vi "element_editor_methane_initial.vi"(9 "Env. Dir":refnum<vi>, 10 "Env. Ready?":refnum<vi>, 11 "Break":refnum<vi>) -> ()   [LabVIEW 2019]
uses:
  lib/libSimulationControl/libSimulationControl.lvlib
panel:
  # "*******************************************************************\nBiogas Plant Control\n\nAuthor: Paul Zügel\nGCSC-Frankfurt am Main 2020\n\n*******************************************************************"
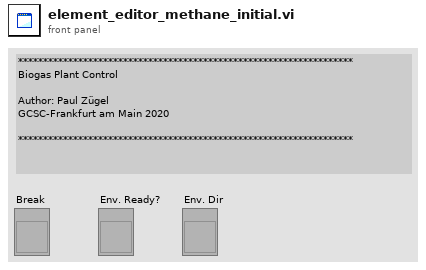
[diagram p1: front panel]
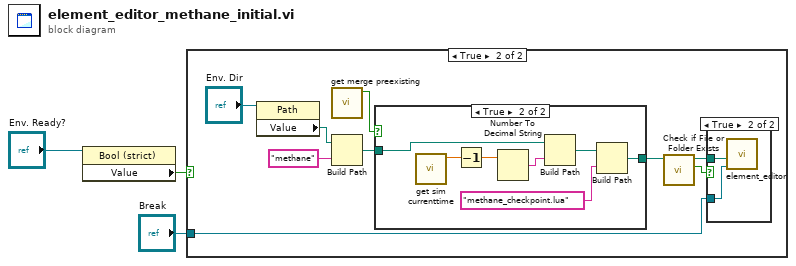
[diagram p0: block diagram]
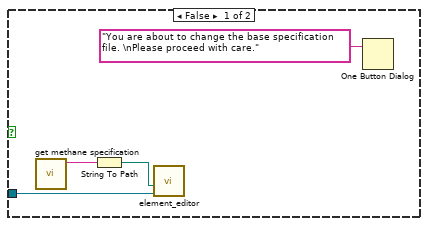
[diagram p2: hidden frame]
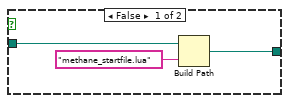
[diagram p3: hidden frame]
diagram:
  n1 = property class="Bool (strict)"(reference="Env. Ready?") -> ("Value"=w1:bool)  [unwired: 1 in, 2 out]
  n2 = case shown="True" w1 {
    tunnel: "Break" -> [w6 w8]
    frame False {
      n3 = call "get methane specification.vi"() -> ("function return"=w5:string)  [unwired: 10 in, 1 out]
      n4 = String To Path(string=w5) -> (path=w4:path)
      n5 = call "element_editor.vi"("Break"=w6, "LUA Specification File"=w4) -> ()  [unwired: 5 in, 1 out]
      n6 = One Button Dialog(message="You are about to change the base specification file. \nPlease proceed with care.") -> ()  [unwired: 1 in, 1 out]
    }
    frame True {
      n7 = property on="Property Node" class="Path"(reference="Env. Dir") -> ("Value"=w15:path)  [unwired: 1 in, 2 out]
      n8 = call "get merge preexisting.vi"() -> ("function return"=w11:bool)  [unwired: 10 in, 1 out]
      n9 = Build Path(base path=w15, name or relative path="methane") -> (appended path=w9:path)
      n10 = case shown="True" w11 {
        tunnel: w9 -> [w18 w26]
        tunnel: [w17 w22] -> w10
        frame False {
          n11 = Build Path(base path=w18, name or relative path="methane_startfile.lua") -> (appended path=w17:path)
        }
        frame True {
          n12 = call "get sim currenttime.vi"() -> ("current_time"=w21:dbl)  [unwired: 10 in, 1 out]
          n13 = Decrement(x=w21) -> (x-1=w20:dbl)
          n14 = Number To Decimal String(number=w20) -> (decimal integer string=w25:string)  [unwired: 1 in]
          n15 = Build Path(base path=w26, name or relative path=w25) -> (appended path=w24:path)
          n16 = Build Path(base path=w24, name or relative path="methane_checkpoint.lua") -> (appended path=w22:path)
        }
      }
      n17 = call <vilib>:"Check if File or Folder Exists.vi"("path"=w10) -> ("file or folder exists?"=w13:bool, "dup path"=w12:path)  [unwired: 8 in, 1 out]
      n18 = case shown="True" w13 {
        tunnel: w12 -> [_ w28]
        tunnel: w8 -> [_ w27]
        frame False {
        }
        frame True {
          n19 = call "element_editor.vi"("Break"=w27, "LUA Specification File"=w28) -> ()  [unwired: 5 in, 1 out]
        }
      }
    }
  }
